vi "Xylo_Essai_3.vi"() -> ()   [LabVIEW 2018]
panel:
  in  "Open Button":bool
  in  "Save As Button":bool
  out "tableauRythme":u8[](array[numeric])
  in  "Rythme Choix":string(combo)
  in  "RESET Button":bool
  out "tableauNotes":u8[](array[numeric])
  in  "stop":bool
  out "Numeric":i32
  in  "Array":bool[](array[boolean])=[FALSE, FALSE, FALSE, FALSE, FALSE, FALSE, FALSE, FALSE] caption="Clavier"
  out "Messure Musicale":dbl(graph)
  in  "File Path Control 2":path
  in  "Save Button":bool
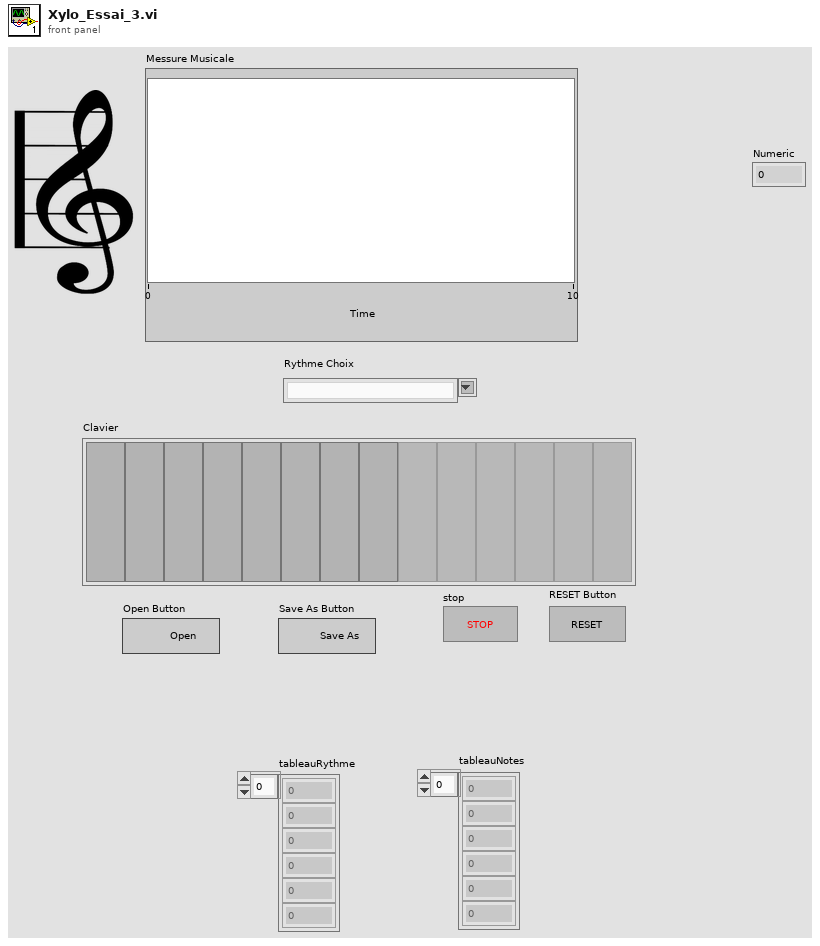
[diagram p1: front panel]
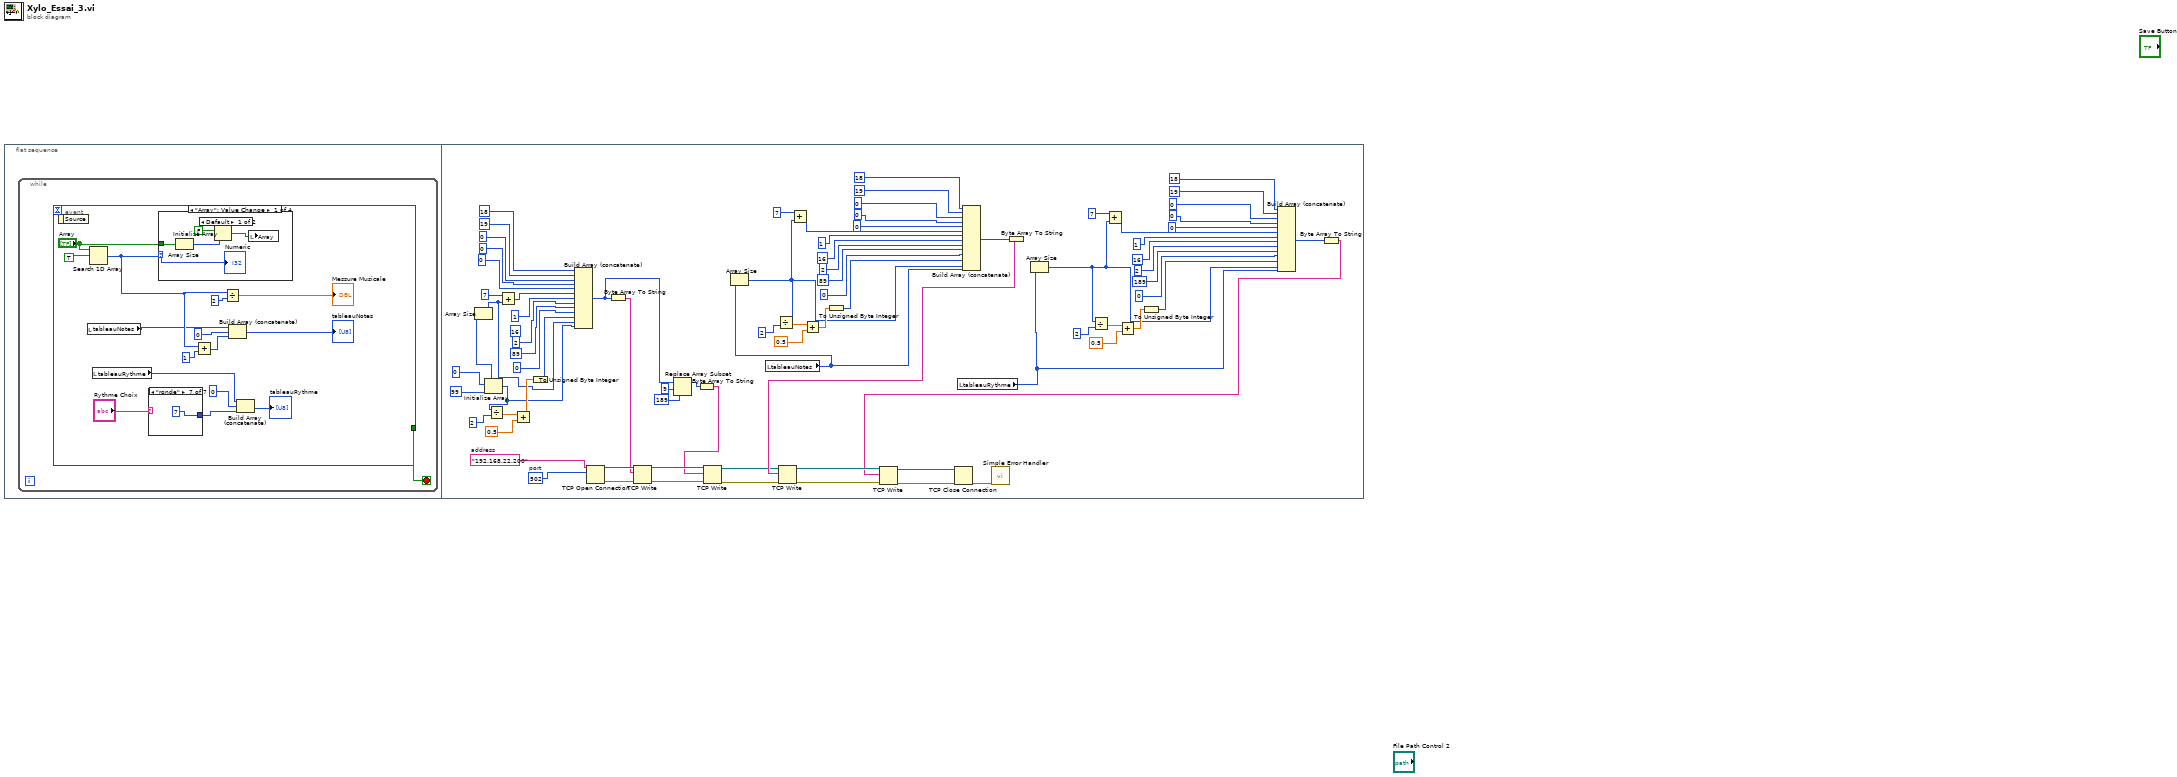
[diagram p0: block diagram]
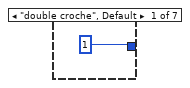
[diagram p2: hidden frame]
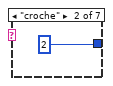
[diagram p3: hidden frame]
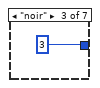
[diagram p4: hidden frame]
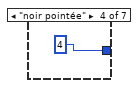
[diagram p5: hidden frame]
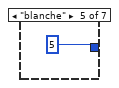
[diagram p6: hidden frame]
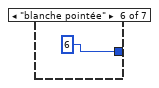
[diagram p7: hidden frame]
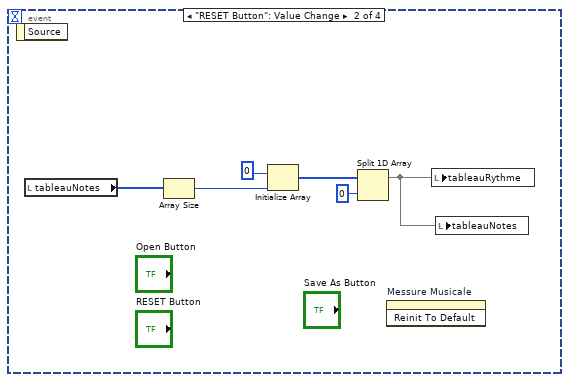
[diagram p9: hidden frame]
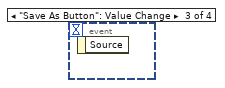
[diagram p10: hidden frame]
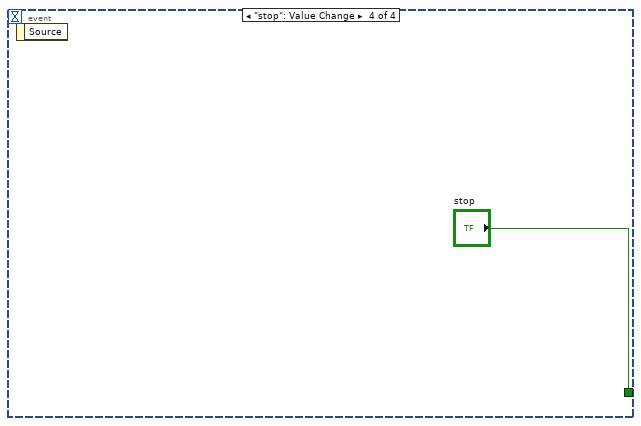
[diagram p11: hidden frame]
diagram:
  n1 = flat-sequence {
    frame #0 {
      n2 = while {
        stop <- w1 stop-if-true
        n3 = event shown="[0] \"Array\": Value Change" {
          selector: _ -> [_ _ _ _]
          dyn-events: _ -> [_ _ _ _]
          timeout: _ -> [_ _ _ _]
          tunnel: [_ _ _ "stop"] -> w1
          event "Array": Value Change {
            n4 = event-data() -> ()  [unwired: 1 in, 1 out]
            n5 = local read "tableauNotes"() -> (w10:u8[])
            n6 = Search 1D Array(1D array="Array", element=TRUE) -> (index of element=w12:i32)  [unwired: 1 in]
            n7 = local read "tableauRythme"() -> (w2:u8[])
            n8 = case shown="\"ronde\"" "Rythme Choix" {
              tunnel: [1 2 3 4 5 6 7] -> w4
              frame "double croche", Default {
              }
              frame "croche" {
              }
              frame "noir" {
              }
              frame "noir pointée" {
              }
              frame "blanche" {
              }
              frame "blanche pointée" {
              }
              frame "ronde" {
              }
            }
            n9 = case shown="Default" w12 {
              selector: w12 -> [w25 _]
              tunnel: "Array" -> [w26 _]
              frame Default {
                n10 = Array Size(array=w26) -> (size(s)=w28:i32)
                n11 = Initialize Array(FALSE ("element"), w28) -> (w24:bool[])
                n12 = local write "Array"(w24) -> ()
                "Numeric" <- w25
              }
              frame -1 {
              }
            }
            n13 = Add(x=w12, y=1) -> (x+y=w9:i32)
            n14 = Divide(x=w12, y=2 ("Numeric")) -> (x/y=→"Messure Musicale":dbl)
            n15 = Build Array (concatenate)(w10, 0 ("element"), w9) -> (→"tableauNotes":i32[])
            n16 = Build Array (concatenate)(w2, 0 ("element"), w4) -> (→"tableauRythme":i32[])
          }
          event "RESET Button": Value Change {
            n17 = event-data() -> ()  [unwired: 1 in, 1 out]
            n18 = local read "tableauNotes"() -> (w33:u8[])
            n19 = Array Size(array=w33) -> (size(s)=w32:i32)
            n20 = Initialize Array(u8 0 ("element"), w32) -> (w31:u8[])
            n21 = Split 1D Array(array=w31, index=0) -> (first subarray=w29:u8[])  [unwired: 1 out]
            n22 = invoke on="Messure Musicale" class="WFChart (strict)" method="Reinit To Default"() -> ()  [unwired: 3 in, 3 out]
            n23 = local write "tableauRythme"(w29) -> ()
            n24 = local write "tableauNotes"(w29) -> ()
          }
          event "Save As Button": Value Change {
            n25 = event-data() -> ()  [unwired: 1 in, 1 out]
          }
          event "stop": Value Change {
            n26 = event-data() -> ()  [unwired: 1 in, 1 out]
          }
        }
      }
    }
    frame #1 {
      (unwired) 16
      w105 = "192.168.22.200"  # address
      w106 = 502  # port
      n27 = Initialize Array(u8 0 ("element"), 99 ("dimension size")) -> (w42:u8[])
      n28 = Array Size(array=w42) -> (size(s)=w43:i32)
      n29 = Divide(x=w42, y=2) -> (x/y=w46:dbl[])
      n30 = Add(x=7, y=w43) -> (x+y=w53:i32)
      n31 = Add(x=w46, y=0.5) -> (x+y=w47:dbl[])
      n32 = To Unsigned Byte Integer(number=w47) -> (unsigned 8bit integer=w44:u8[])
      n33 = Build Array (concatenate)(18, 19, 0, 0, 0, w53, 1, 2, 89, 0, w44, w43, w42) -> (w40:i32[])
      n34 = TCP Open Connection(address=w105, remote port or service name=w106) -> (connection ID=w67:refnum<k5>, error out=w64:errorcluster)  [unwired: 3 in]
      n35 = Byte Array To String(unsigned byte array=w40) -> (string=w41:string)
      n36 = TCP Write(connection ID=w67, data in=w41, error in (no error)=w64) -> (connection ID out=w66:refnum<k5>, error out=w63:errorcluster)  [unwired: 1 in, 1 out]
      n37 = Replace Array Subset(array=w40, new element=189 ("new element/subarray"), index=9) -> (w37:i32[])
      n38 = Byte Array To String(unsigned byte array=w37) -> (string=w36:string)
      n39 = TCP Write(connection ID=w66, data in=w36, error in (no error)=w63) -> (connection ID out=w65:refnum<k5>, error out=w62:errorcluster)  [unwired: 1 in, 1 out]
      n40 = local read "tableauNotes"() -> (w97:u8[])
      n41 = Array Size(array=w97) -> (size(s)=w94:i32)
      n42 = Divide(x=w94, y=2) -> (x/y=w95:dbl)
      n43 = Add(x=7, y=w94) -> (x+y=w116:i32)
      n44 = Add(x=w95, y=0.5) -> (x+y=w103:dbl)
      n45 = To Unsigned Byte Integer(number=w103) -> (unsigned 8bit integer=w98:u8)
      n46 = local read "tableauRythme"() -> (w69:u8[])
      n47 = Build Array (concatenate)(18, 19, 0, 0, 0, w116, 1, 16, 2, 89, 0, w98, w94, w97) -> (w115:i32[])
      n48 = Byte Array To String(unsigned byte array=w115) -> (string=w114:string)
      n49 = TCP Write(connection ID=w65, data in=w114, error in (no error)=w62) -> (connection ID out=w92:refnum<k5>, error out=w91:errorcluster)  [unwired: 1 in, 1 out]
      n50 = Array Size(array=w69) -> (size(s)=w71:i32)
      n51 = Divide(x=w71, y=2) -> (x/y=w72:dbl)
      n52 = Add(x=7, y=w71) -> (x+y=w88:i32)
      n53 = Add(x=w72, y=0.5) -> (x+y=w79:dbl)
      n54 = To Unsigned Byte Integer(number=w79) -> (unsigned 8bit integer=w74:u8)
      n55 = Build Array (concatenate)(18, 19, 0, 0, 0, w88, 1, 16, 2, 189, 0, w74, w71, w69) -> (w87:i32[])
      n56 = Byte Array To String(unsigned byte array=w87) -> (string=w68:string)
      n57 = TCP Write(connection ID=w92, data in=w68, error in (no error)=w91) -> (connection ID out=w89:refnum<k5>, error out=w90:errorcluster)  [unwired: 1 in, 1 out]
      n58 = TCP Close Connection(connection ID=w89, error in (no error)=w90) -> (error out=w113:errorcluster)  [unwired: 1 in, 1 out]
      n59 = call <vilib>:"Simple Error Handler.vi"("error in (no error)"=w113) -> ()  [unwired: 4 in, 5 out]
    }
  }
